vi "Get Channel References.vi"(8 "error in (no error)":errorcluster, 11 "Item Ref in":T1 format="%.0x") -> (0 "error out":errorcluster, 2 "Channel Refs out":T1[](array[typedef]) format="%.0x", 3 "Item Ref out":T1 format="%.0x")   [LabVIEW 2027, in "System Monitor System Explorer.lvlib"]
uses:
  System Monitor System Explorer.lvlib
  <vilib>/NI VeriStand/Custom Device API/Custom Device Item Ref.ctl
  <vilib>/NI VeriStand/Custom Device API/Custom Device API.lvlib
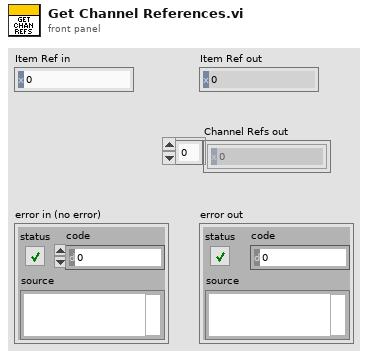
[diagram p1: front panel]
types:
  T1 = typedef "Custom Device API.lvlib/Custom Device Item Ref.ctl" = u64
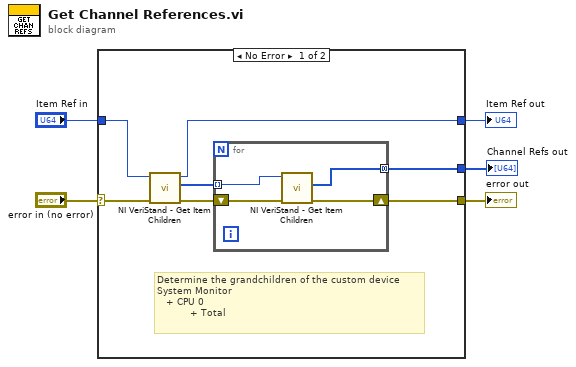
[diagram p0: block diagram]
diagram:
  n1 = case shown="No Error" "error in (no error)" {
    selector: "error in (no error)" -> [w7 w18]
    tunnel: [w11 w18] -> w5
    tunnel: [w10 w17] -> w4
    tunnel: "Item Ref in" -> [w8 w17]
    tunnel: [w6 _] -> w1
    frame No Error {
      # "Determine the grandchildren of the custom device\nSystem Monitor\n   + CPU 0\n           + Total"
      n2 = call <vilib>:"NI VeriStand - Get Item Children.vi"("error in (no error)"=w7, "Item Ref in"=w8) -> ("error out"=w9:errorcluster, "Child Refs"=w12:T1[], "Item Ref out"=w10:T1)  [unwired: 6 in, 1 out]
      n3 = for {
        shift-right: [w15] -> w11
        shift-left: w9 -> [w16]
        tunnel: w12 -> [w14] mode=indexing
        tunnel: [w13] -> w6 mode=concatenating
        n4 = call <vilib>:"NI VeriStand - Get Item Children.vi"("error in (no error)"=w16, "Item Ref in"=w14) -> ("error out"=w15:errorcluster, "Child Refs"=w13:T1[])  [unwired: 6 in, 2 out]
      }
    }
    frame Error {
    }
  }
  "error out" <- w5
  "Item Ref out" <- w4
  "Channel Refs out" <- w1
